vi "GetAllSeries.vi"() -> ()   [LabVIEW 2024]
uses:
  <vilib>/addons/_JKI.lib/REST Client/classes/REST Client/REST Client.lvclass
panel:
  in  "Stop":bool
  out "last offset":i32
  out "progress":i32(slide) caption="2110 of 5155" scale=0.0..5155.0
  in  "series offset":i32
  in  "Number of Series to GET":i32
  out "error out":errorcluster
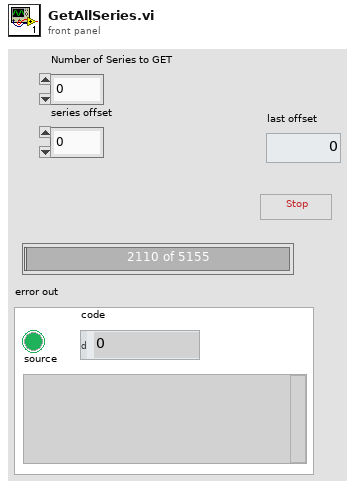
[diagram p1: front panel]
types:
  T1 = typedef "series.reply.ctl" = cluster{"code":i32, "status":string, "etag":string, "data":cluster{"offset":i32, "limit":i32, "total":i32, "count":i32, "results":cluster{"id":i32, "title":string, "description":string, "resourceURI":string, "urls":cluster{"type":string, "url":string}[], "startYear":i32, "endYear":i32, "rating":string, "type":string, "modified":variant, "thumbnail":cluster{"path":string, "extension":string}, "creators":cluster{"available":i32, "returned":i32, "collectionURI":string, "items":cluster{"resourceURI":string, "name":string, "role":string}[]}, "comics":cluster{"available":i32, "returned":i32, "collectionURI":string, "items":cluster{"resourceURI":string, "name":string}[]}, "characters":cluster{"available":i32, "returned":i32, "collectionURI":string, "items":cluster{"resourceURI":string, "name":string}[]}, "stories":cluster{"available":i32, "returned":i32, "collectionURI":string, "items":cluster{"resourceURI":string, "name":string, "type":string}[]}, "events":cluster{"available":i32, "returned":i32, "collectionURI":string, "items":cluster{"resourceURI":string, "name":string}[]}, "next":variant, "previous":variant}[]}}
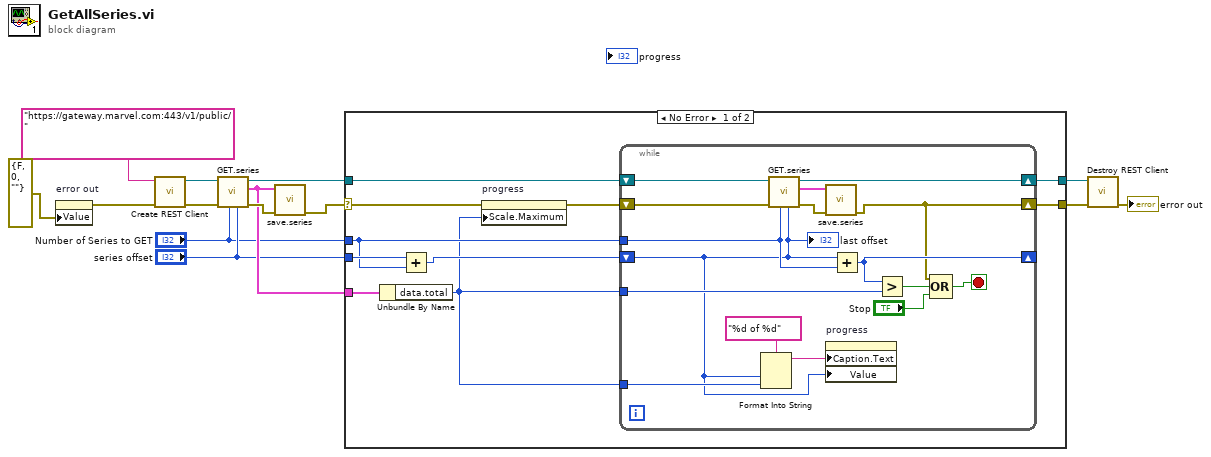
[diagram p0: block diagram]
diagram:
  n1 = property on="error out" class="Clust (strict)"("Value"=errorcluster {"status"=FALSE, "code"=0, "source"=""} ("error out")) -> (error out=w2:errorcluster)  [unwired: 2 in, 1 out]
  n2 = call <vilib>:"Create REST Client.vi"("error in (no error)"=w2, "Base URL"="https://gateway.marvel.com:443/v1/public/") -> ("error out"=w12:errorcluster, "REST Client out"=w13:refnum<class "REST Client.lvclass">)  [unwired: 8 in]
  n3 = call "GET.series.vi"("series offset"="series offset", "Number of Series to GET"="Number of Series to GET", "error in (no error)"=w12, "REST Client in"=w13) -> ("error out"=w10:errorcluster, "data"=w9:T1, "REST Client out"=w8:refnum<class "REST Client.lvclass">)  [unwired: 5 in]
  n4 = call "save.series.vi"("error in"=w10, "data"=w9) -> ("error out"=w3:errorcluster)  [unwired: 9 in]
  n5 = case shown="No Error" w3 {
    selector: w3 -> [w15 w41]
    tunnel: w9 -> [w24 _]
    tunnel: w8 -> [w23 w42]
    tunnel: [w22 w42] -> w7
    tunnel: [w21 w41] -> w6
    tunnel: "series offset" -> [w20 _]
    tunnel: "Number of Series to GET" -> [w19 _]
    frame No Error {
      n6 = Unbundle By Name(w24) -> ("data.total"=w16:i32)
      n7 = Add(x=w20, y=w19) -> (x+y=w18:i32)
      n8 = property on="progress" class="Slide (strict)"(error in=w15, "Scale.Maximum"=w16) -> (error out=w17:errorcluster)  [unwired: 1 in, 1 out]
      n9 = while {
        shift-right: [w37] -> w22
        shift-left: w23 -> [w38]
        shift-right: [w31] -> w21
        shift-left: w17 -> [w36]
        tunnel: w19 -> [w35]
        shift-right: [w34] -> _
        shift-left: w18 -> [w26]
        tunnel: w16 -> [w33]
        tunnel: w16 -> [w28]
        stop <- w30 stop-if-true
        n10 = Format Into String(format string="%d of %d", w26, w28) -> (resulting string=w27:string)  [unwired: 2 in, 1 out]
        n11 = call "GET.series.vi"("series offset"=w26, "Number of Series to GET"=w35, "error in (no error)"=w36, "REST Client in"=w38) -> ("error out"=w39:errorcluster, "data"=w40:T1, "REST Client out"=w37:refnum<class "REST Client.lvclass">)  [unwired: 5 in]
        n12 = call "save.series.vi"("error in"=w39, "data"=w40) -> ("error out"=w31:errorcluster)  [unwired: 9 in]
        n13 = property on="progress" class="Slide (strict)"("Caption.Text"=w27, "Value"=w26) -> ()  [unwired: 2 in, 2 out]
        n14 = Add(x=w26, y=w35) -> (x+y=w34:i32)
        n15 = Greater?(x=w34, y=w33) -> (0:w32:bool)
        n16 = Compound Arithmetic op=OR(w31, w32, "Stop") -> (w30:bool)
        "last offset" <- w26
      }
    }
    frame Error {
    }
  }
  n17 = call-dynamic "Destroy REST Client.vi"("error in (no error)"=w6, "REST Client in"=w7) -> ("error out"=→"error out":errorcluster)  [unwired: 9 in]
